vi "Drive over defenses.vi"(8 "Type of Defense":T1(ring), 10 "navX Device":T2 {"Interface"."Update Rate (4Hz-60Hz)" min=4 max=60 step=1}, 11 "RobotDriveDevRef":T4) -> ()   [LabVIEW 2015]
uses:
  <vilib>/Rock Robotics/WPI/RobotDrive/WPI_RobotDriveDevRef.ctl
  <vilib>/Rock Robotics/WPI/MotorControl/WPI_MotorControlDeviceRef.ctl
  <vilib>/Rock Robotics/WPI/MotorControl/WPI_MotorControlType.ctl
  <vilib>/Rock Robotics/SystemInterfaces/DIO/FPGA_DIOPWMChannel.ctl
  <vilib>/Rock Robotics/WPI/PWM/WPI_PWMDeadband.ctl
  <vilib>/Rock Robotics/WPI/CAN/Jaguar/SubVIs/WPI_CANJaguar_ControlMode.ctl
  <vilib>/Rock Robotics/WPI/CAN/TalonSRX/WPI_CANTalonSRX_APIControlMode.ctl
  navx-mxp/labview/navX Library v2/TypeDefs/Z900_navX_DeviceTypeDef.ctl
  navx-mxp/labview/navX Library v2/TypeDefs/Z900_navX_ProtocolTypeDef.ctl
  navx-mxp/labview/navX Library v2/TypeDefs/Z900_navX_NotifyPacketTypeDef.ctl
  navx-mxp/labview/navX Library v2/TypeDefs/Z900_navX_ActionTypeDef.ctl
  <vilib>/Rock Robotics/WPI/RobotDrive/WPI_RobotDriveArcadeDrive_Standard(NoSaturation).vi
  navx-mxp/labview/navX Library v2/navX Library v2.lvlib
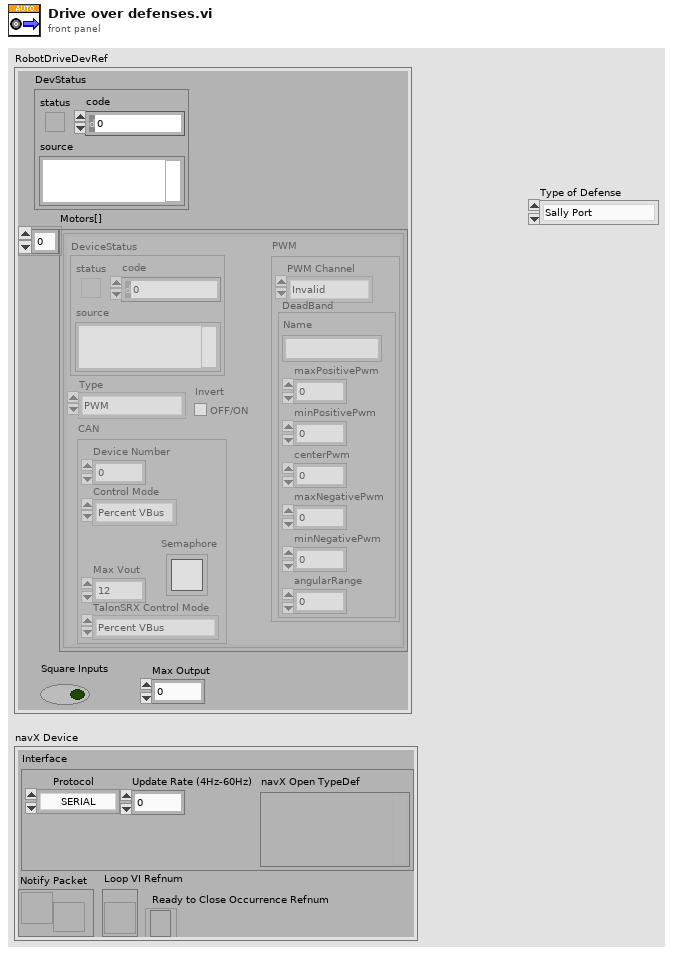
[diagram p1: front panel]
types:
  T1 = enum16{"Sally Port", "Portcullis", "Drawbridge", "Moat", "Rock Wall", "Cheval De Frise", "Ramparts", "Low Bar", "Rocky Terrain"}
  T2 = typedef "navX Library v2.lvlib/Z900_navX_DeviceTypeDef.ctl" = cluster{"Interface":cluster{"Protocol":T3, "Update Rate (4Hz-60Hz)":u8, "navX Open TypeDef":variant}, "Notify Packet":refnum<notifier>, "Loop VI Refnum":refnum<vi>, "Ready to Close Occurrence Refnum":refnum<k4>}
  T3 = typedef "navX Library v2.lvlib/Z900_navX_ProtocolTypeDef.ctl" = enum16{"SERIAL", "I2C", "SPI"}
  T4 = typedef "WPI_RobotDriveDevRef.ctl" = cluster{"DevStatus":errorcluster, "Motors[]":T5[], "Square Inputs":bool, "Max Output":dbl}
  T5 = typedef "WPI_MotorControlDeviceRef.ctl" = cluster{"DeviceStatus":errorcluster, "Type":T6, "PWM":cluster{"PWM Channel":T7, "DeadBand":T8}, "CAN":cluster{"Device Number":u8, "Control Mode":T9, "Semaphore":T10, "Max Vout":dbl, "TalonSRX Control Mode":T11}, "Invert":bool}
  T6 = typedef "WPI_MotorControlType.ctl" = enum16{"PWM", "CAN", "CANTalonSRX"}
  T7 = typedef "FPGA_DIOPWMChannel.ctl" = enum8{"PWM 0", "PWM 1", "PWM 2", "PWM 3", "PWM 4", "PWM 5", "PWM 6", "PWM 7", "PWM 8", "PWM 9", "PWM MXP 0", "PWM MXP 1", "PWM MXP 2", "PWM MXP 3", "PWM MXP 4", "PWM MXP 5", "PWM MXP 6", "PWM MXP 7", "PWM MXP 8", "PWM MXP 9", "Invalid"}
  T8 = typedef "WPI_PWMDeadband.ctl" = cluster{"Name":string, "maxPositivePwm":i32, "minPositivePwm":i32, "centerPwm":i32, "maxNegativePwm":i32, "minNegativePwm":i32, "angularRange":u16}
  T9 = typedef "WPI_CANJaguar_ControlMode.ctl" = enum8{"Percent VBus", "Current", "Speed", "Position", "Voltage"}
  T10 = typedef "Semaphore RefNum" = refnum<k1>
  T11 = typedef "WPI_CANTalonSRX_APIControlMode.ctl" = enum8{"Percent VBus", "Speed", "Position", "Slave", "Unchanged / Invalid", "Voltage Compensation", "Current", "Motion Profile"}
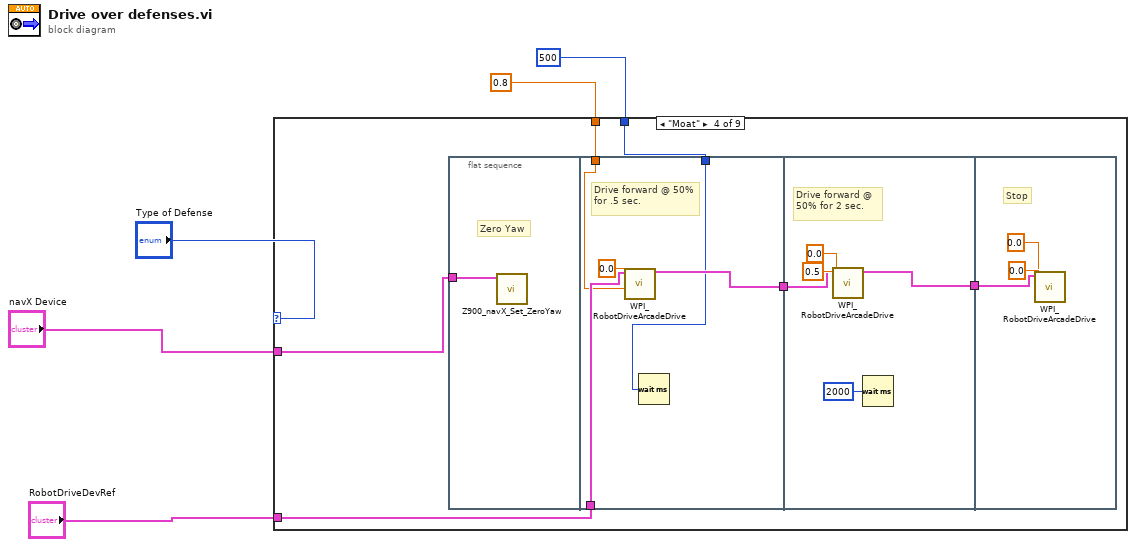
[diagram p0: block diagram]
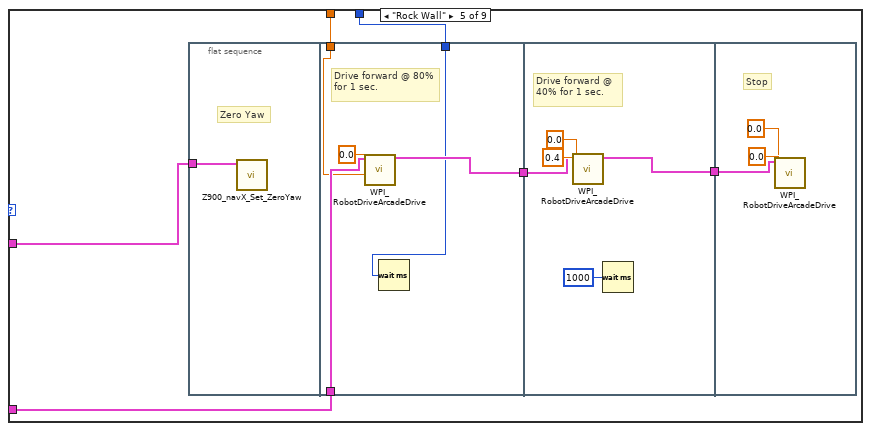
[diagram p5: hidden frame]
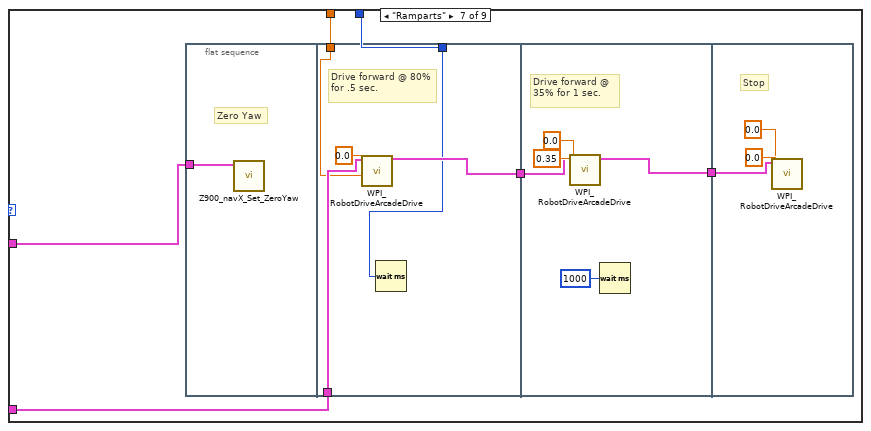
[diagram p7: hidden frame]
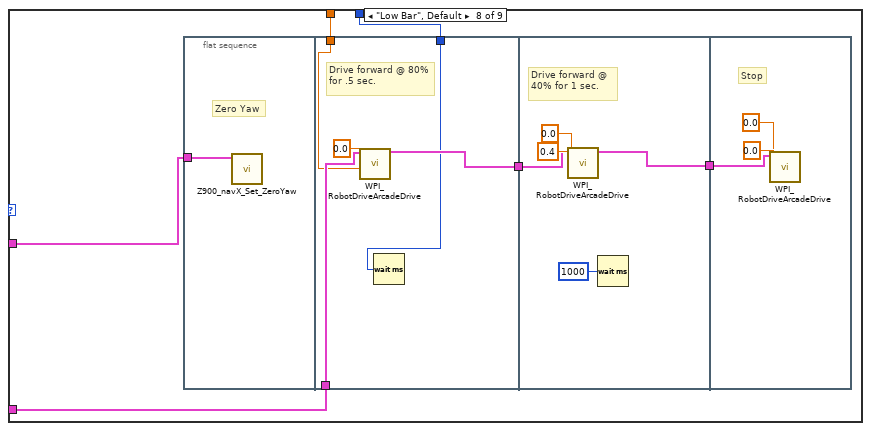
[diagram p8: hidden frame]
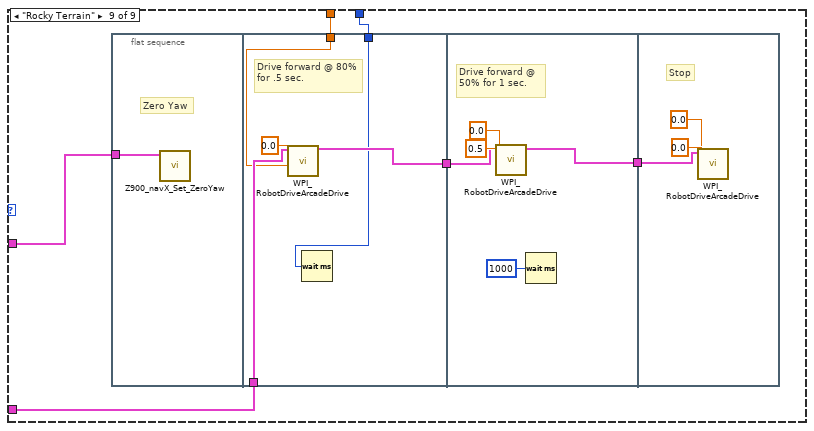
[diagram p9: hidden frame]
diagram:
  n1 = case shown="\"Moat\"" "Type of Defense" {
    tunnel: "RobotDriveDevRef" -> [_ _ _ w8 w28 _ w48 w68 w88]
    tunnel: "navX Device" -> [_ _ _ w9 w29 _ w49 w69 w89]
    tunnel: 0.8 ("Y axis value") -> [_ _ _ w7 w27 _ w47 w67 w87]
    tunnel: u32 500 ("milliseconds to wait") -> [_ _ _ w6 w26 _ w46 w66 w86]
    frame "Sally Port" {
    }
    frame "Portcullis" {
    }
    frame "Drawbridge" {
    }
    frame "Moat" {
      n2 = flat-sequence {
        tunnel: w9 -> [w12]
        tunnel: [w16] -> w11
        tunnel: w8 -> [w15]
        tunnel: w7 -> [w14]
        tunnel: w6 -> [w13]
        tunnel: w11 -> [w20]
        tunnel: [w19] -> w10
        tunnel: w10 -> [w23]
        frame #0 {
          # "Zero Yaw"
          n3 = call "Z900_navX_Set_ZeroYaw.vi"("navX Device"=w12) -> ()  [unwired: 9 in, 2 out]
        }
        frame #1 {
          # "Drive forward @ 50% for .5 sec."
          n4 = call-poly <vilib>:"WPI_RobotDriveArcadeDrive.vi"("Y axis value"=w14, "X axis value"=0.0, "RobotDriveDevRef"=w15) -> ("RobotDriveDevRef"=w16:T4)  [unwired: 6 in, 2 out]
          n5 = Wait (ms)(milliseconds to wait=w13) -> ()  [unwired: 1 out]
        }
        frame #2 {
          # "Drive forward @ 50% for 2 sec."
          n6 = call-poly <vilib>:"WPI_RobotDriveArcadeDrive.vi"("Y axis value"=0.5, "X axis value"=0.0, "RobotDriveDevRef"=w20) -> ("RobotDriveDevRef"=w19:T4)  [unwired: 6 in, 2 out]
          n7 = Wait (ms)(milliseconds to wait=u32 2000) -> ()  [unwired: 1 out]
        }
        frame #3 {
          # "Stop"
          n8 = call-poly <vilib>:"WPI_RobotDriveArcadeDrive.vi"("Y axis value"=0.0, "X axis value"=0.0, "RobotDriveDevRef"=w23) -> ()  [unwired: 6 in, 3 out]
        }
      }
    }
    frame "Rock Wall" {
      n9 = flat-sequence {
        tunnel: w29 -> [w32]
        tunnel: [w36] -> w31
        tunnel: w28 -> [w35]
        tunnel: w27 -> [w34]
        tunnel: w26 -> [w33]
        tunnel: w31 -> [w40]
        tunnel: [w39] -> w30
        tunnel: w30 -> [w43]
        frame #0 {
          # "Zero Yaw"
          n10 = call "Z900_navX_Set_ZeroYaw.vi"("navX Device"=w32) -> ()  [unwired: 9 in, 2 out]
        }
        frame #1 {
          # "Drive forward @ 80% for 1 sec."
          n11 = call-poly <vilib>:"WPI_RobotDriveArcadeDrive.vi"("Y axis value"=w34, "X axis value"=0.0, "RobotDriveDevRef"=w35) -> ("RobotDriveDevRef"=w36:T4)  [unwired: 6 in, 2 out]
          n12 = Wait (ms)(milliseconds to wait=w33) -> ()  [unwired: 1 out]
        }
        frame #2 {
          # "Drive forward @ 40% for 1 sec."
          n13 = call-poly <vilib>:"WPI_RobotDriveArcadeDrive.vi"("Y axis value"=0.4, "X axis value"=0.0, "RobotDriveDevRef"=w40) -> ("RobotDriveDevRef"=w39:T4)  [unwired: 6 in, 2 out]
          n14 = Wait (ms)(milliseconds to wait=u32 1000) -> ()  [unwired: 1 out]
        }
        frame #3 {
          # "Stop"
          n15 = call-poly <vilib>:"WPI_RobotDriveArcadeDrive.vi"("Y axis value"=0.0, "X axis value"=0.0, "RobotDriveDevRef"=w43) -> ()  [unwired: 6 in, 3 out]
        }
      }
    }
    frame "Cheval De Frise" {
    }
    frame "Ramparts" {
      n16 = flat-sequence {
        tunnel: w49 -> [w52]
        tunnel: [w56] -> w51
        tunnel: w48 -> [w55]
        tunnel: w47 -> [w54]
        tunnel: w46 -> [w53]
        tunnel: w51 -> [w60]
        tunnel: [w59] -> w50
        tunnel: w50 -> [w63]
        frame #0 {
          # "Zero Yaw"
          n17 = call "Z900_navX_Set_ZeroYaw.vi"("navX Device"=w52) -> ()  [unwired: 9 in, 2 out]
        }
        frame #1 {
          # "Drive forward @ 80% for .5 sec."
          n18 = call-poly <vilib>:"WPI_RobotDriveArcadeDrive.vi"("Y axis value"=w54, "X axis value"=0.0, "RobotDriveDevRef"=w55) -> ("RobotDriveDevRef"=w56:T4)  [unwired: 6 in, 2 out]
          n19 = Wait (ms)(milliseconds to wait=w53) -> ()  [unwired: 1 out]
        }
        frame #2 {
          # "Drive forward @ 35% for 1 sec."
          n20 = call-poly <vilib>:"WPI_RobotDriveArcadeDrive.vi"("Y axis value"=0.35, "X axis value"=0.0, "RobotDriveDevRef"=w60) -> ("RobotDriveDevRef"=w59:T4)  [unwired: 6 in, 2 out]
          n21 = Wait (ms)(milliseconds to wait=u32 1000) -> ()  [unwired: 1 out]
        }
        frame #3 {
          # "Stop"
          n22 = call-poly <vilib>:"WPI_RobotDriveArcadeDrive.vi"("Y axis value"=0.0, "X axis value"=0.0, "RobotDriveDevRef"=w63) -> ()  [unwired: 6 in, 3 out]
        }
      }
    }
    frame "Low Bar", Default {
      n23 = flat-sequence {
        tunnel: w69 -> [w72]
        tunnel: [w76] -> w71
        tunnel: w68 -> [w75]
        tunnel: w67 -> [w74]
        tunnel: w66 -> [w73]
        tunnel: w71 -> [w80]
        tunnel: [w79] -> w70
        tunnel: w70 -> [w83]
        frame #0 {
          # "Zero Yaw"
          n24 = call "Z900_navX_Set_ZeroYaw.vi"("navX Device"=w72) -> ()  [unwired: 9 in, 2 out]
        }
        frame #1 {
          # "Drive forward @ 80% for .5 sec."
          n25 = call-poly <vilib>:"WPI_RobotDriveArcadeDrive.vi"("Y axis value"=w74, "X axis value"=0.0, "RobotDriveDevRef"=w75) -> ("RobotDriveDevRef"=w76:T4)  [unwired: 6 in, 2 out]
          n26 = Wait (ms)(milliseconds to wait=w73) -> ()  [unwired: 1 out]
        }
        frame #2 {
          # "Drive forward @ 40% for 1 sec."
          n27 = call-poly <vilib>:"WPI_RobotDriveArcadeDrive.vi"("Y axis value"=0.4, "X axis value"=0.0, "RobotDriveDevRef"=w80) -> ("RobotDriveDevRef"=w79:T4)  [unwired: 6 in, 2 out]
          n28 = Wait (ms)(milliseconds to wait=u32 1000) -> ()  [unwired: 1 out]
        }
        frame #3 {
          # "Stop"
          n29 = call-poly <vilib>:"WPI_RobotDriveArcadeDrive.vi"("Y axis value"=0.0, "X axis value"=0.0, "RobotDriveDevRef"=w83) -> ()  [unwired: 6 in, 3 out]
        }
      }
    }
    frame "Rocky Terrain" {
      n30 = flat-sequence {
        tunnel: w89 -> [w92]
        tunnel: [w96] -> w91
        tunnel: w88 -> [w95]
        tunnel: w87 -> [w94]
        tunnel: w86 -> [w93]
        tunnel: w91 -> [w100]
        tunnel: [w99] -> w90
        tunnel: w90 -> [w103]
        frame #0 {
          # "Zero Yaw"
          n31 = call "Z900_navX_Set_ZeroYaw.vi"("navX Device"=w92) -> ()  [unwired: 9 in, 2 out]
        }
        frame #1 {
          # "Drive forward @ 80% for .5 sec."
          n32 = call-poly <vilib>:"WPI_RobotDriveArcadeDrive.vi"("Y axis value"=w94, "X axis value"=0.0, "RobotDriveDevRef"=w95) -> ("RobotDriveDevRef"=w96:T4)  [unwired: 6 in, 2 out]
          n33 = Wait (ms)(milliseconds to wait=w93) -> ()  [unwired: 1 out]
        }
        frame #2 {
          # "Drive forward @ 50% for 1 sec."
          n34 = call-poly <vilib>:"WPI_RobotDriveArcadeDrive.vi"("Y axis value"=0.5, "X axis value"=0.0, "RobotDriveDevRef"=w100) -> ("RobotDriveDevRef"=w99:T4)  [unwired: 6 in, 2 out]
          n35 = Wait (ms)(milliseconds to wait=u32 1000) -> ()  [unwired: 1 out]
        }
        frame #3 {
          # "Stop"
          n36 = call-poly <vilib>:"WPI_RobotDriveArcadeDrive.vi"("Y axis value"=0.0, "X axis value"=0.0, "RobotDriveDevRef"=w103) -> ()  [unwired: 6 in, 3 out]
        }
      }
    }
  }
